vi "Write User Status.vi"(8 "error in (no error)":errorcluster, 10 "User Status":bool, 11 "Session in":refnum<class "Session.lvclass">) -> (0 "error out":errorcluster, 3 "Session out":refnum<class "Session.lvclass">)   [LabVIEW 2024, in "CTI.lvlib" / "Session.lvclass"]
doc: "Specifies whether the status LED is lit or off. Calling this VI automatically puts the Status Source into User mode and the status LED will remain in the set state until changed by calling this VI again or changing the status source with <b>Write Status Source.vi</b>."
uses:
  Session.lvclass
  DeviceComms/DeviceComms.lvclass
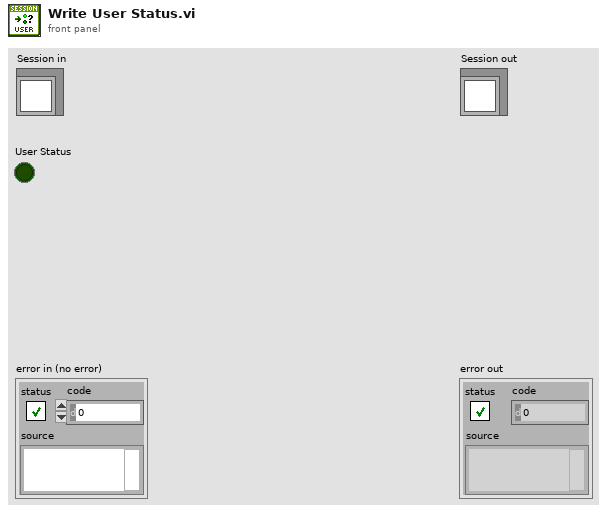
[diagram p1: front panel]
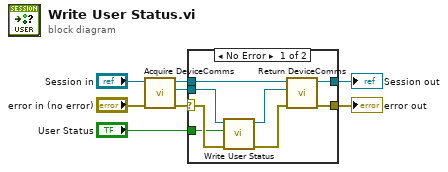
[diagram p0: block diagram]
diagram:
  n1 = call "Acquire DeviceComms.vi"("error in (no error)"="error in (no error)", "Session in"="Session in") -> ("error out"=w8:errorcluster, "DeviceComms"=w4:refnum<class "DeviceComms.lvclass">, "Session out"=w5:refnum<class "Session.lvclass">)  [unwired: 7 in]
  n2 = case shown="No Error" w8 {
    selector: w8 -> [w16 w17]
    tunnel: w5 -> [w15 w18]
    tunnel: w4 -> [w14 _]
    tunnel: "User Status" -> [w13 _]
    tunnel: [w12 w18] -> w2
    tunnel: [w9 w17] -> w1
    frame No Error {
      n3 = call-dynamic "Write User Status.vi"("error in (no error)"=w16, "User Status"=w13, "DeviceComms in"=w14) -> ("error out"=w10:errorcluster, "DeviceComms out"=w11:refnum<class "DeviceComms.lvclass">)  [unwired: 7 in]
      n4 = call "Return DeviceComms.vi"("error in (no error)"=w10, "DeviceComms"=w11, "Session in"=w15) -> ("error out"=w9:errorcluster, "Session out"=w12:refnum<class "Session.lvclass">)  [unwired: 7 in]
    }
    frame Error {
    }
  }
  "error out" <- w1
  "Session out" <- w2
